vi "Reset.vi"(8 "error in (no error)":errorcluster, 9 "command":u8(ring)=5 items=["reset counter value"=1, "reset alarm"=2, "restart batch counter"=3, "reset counter value (counter off)"=4, "reset module"=5], 10 "node address (same)":u8, 11 "ProPar in":refnum<class "PL Bronkhorst ProPar.lvclass">) -> (0 "error out":errorcluster, 3 "ProPar out":refnum<class "PL Bronkhorst ProPar.lvclass">)   [LabVIEW 2015, in "PL Bronkhorst ProPar.lvclass"]
doc: "Resets specified <b>node</b>."
uses:
  PL Bronkhorst ProPar.lvclass
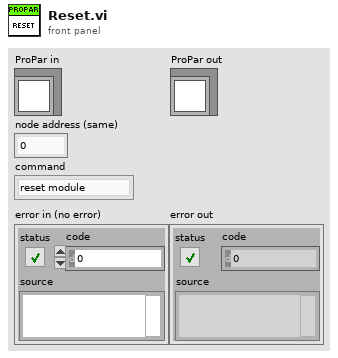
[diagram p1: front panel]
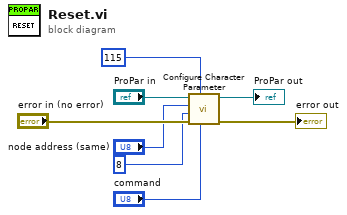
[diagram p0: block diagram]
diagram:
  n1 = call "Configure Character Parameter.vi"("value"="command", "process number"=u8 115, "error in (no error)"="error in (no error)", "parameter number"=u8 8 ("process number"), "node address (same)"="node address (same)", "ProPar in"="ProPar in") -> ("error out"=→"error out":errorcluster, "ProPar out"=→"ProPar out":refnum<class "PL Bronkhorst ProPar.lvclass">)  [unwired: 4 in]
